vi "WriteTracepoints.vi"(8 "error in (no error)":errorcluster, 11 "log dir":path) -> (0 "error out":errorcluster, 3 "tracepoints":T1[](array[typedef]))   [LabVIEW 2017, in "TraceLogger.lvlib"]
uses:
  <vilib>/addons/TraceLogger/TraceLogger.lvlib
  <vilib>/addons/TraceLogger/controls/TracepointConfig.ctl
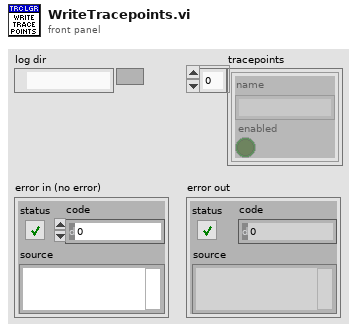
[diagram p1: front panel]
types:
  T1 = typedef "TraceLogger.lvlib/TracepointConfig.ctl" = cluster{"name":string, "enabled":bool}
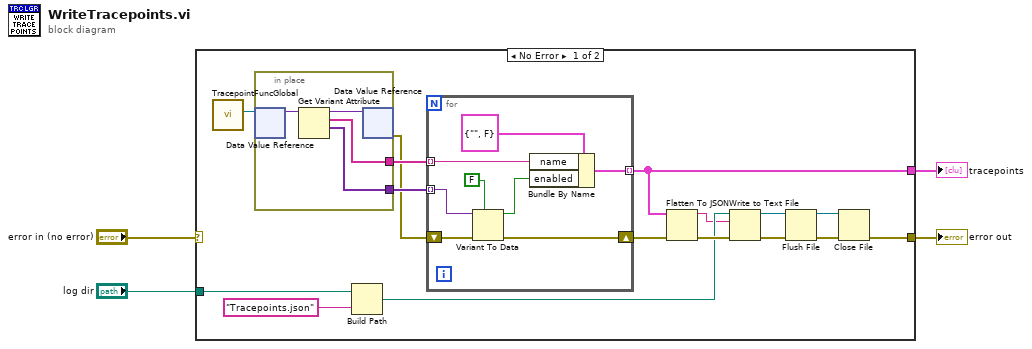
[diagram p0: block diagram]
diagram:
  n1 = case shown="No Error" "error in (no error)" {
    selector: "error in (no error)" -> [_ w33]
    tunnel: [w9 w33] -> w4
    tunnel: "log dir" -> [w19 _]
    tunnel: [w10 _] -> w1
    frame No Error {
      n2 = call <vilib>:"TracepointFuncGlobal.vi"() -> ("tracepoints"=w18:refnum<data-value>)  [unwired: 11 in]
      n3 = in-place {
        in-place-border: [w22] -> w17
        in-place-border: [w21] -> w16
        n4 = in-place-dvr #1(w18) -> (w24:variant)  [unwired: 1 out]
        n5 = Get Variant Attribute(Variant=w24) -> (duplicate Variant=w23:variant, names=w22:string[], values=w21:variant[])  [unwired: 3 in, 1 out]
        n6 = in-place-dvr #1(w23) -> (w15:errorcluster)  [unwired: 1 out]
      }
      n7 = Build Path(base path=w19, name or relative path="Tracepoints.json") -> (appended path=w12:path)
      n8 = for {
        tunnel: w17 -> [w31] mode=indexing
        tunnel: w16 -> [w30] mode=indexing
        tunnel: [w27] -> w10 mode=indexing
        shift-right: [w25] -> w14
        shift-left: w15 -> [w26]
        n9 = Variant To Data(error in=w26, type=FALSE, Variant=w30) -> (data=w28:bool, error out=w25:errorcluster)
        n10 = Bundle By Name(cluster=T1 {"name"="", "enabled"=FALSE} ("TracePoint"), "name"=w31, "enabled"=w28) -> (w27:T1)
      }
      n11 = Flatten To JSON(anything=w10, error in (no error)=w14) -> (JSON string=w11:string, 11:w13:errorcluster)  [unwired: 1 in]
      n12 = Write to Text File(file (use dialog)=w12, text=w11, error in=w13) -> (refnum out=w8:refnum<file>, error out=w6:errorcluster)  [unwired: 1 in, 1 out]
      n13 = Flush File(refnum=w8, error in=w6) -> (refnum out=w7:refnum<file>, error out=w5:errorcluster)
      n14 = Close File(refnum=w7, error in=w5) -> (error out=w9:errorcluster)  [unwired: 1 out]
    }
    frame Error {
    }
  }
  "error out" <- w4
  "tracepoints" <- w1
